vi "tm3samp_07b_dcimgrecorder_wVision.vi"() -> ()   [LabVIEW 2023]
panel:
  out "Frames Recorded":i32
  in  "Frames":i32=100
  in  "DCIMG Path":path
  out "Display":T1(plugin-control)
  out "DCAM Version":string
  out "Library Version":string
  out "Error Out":errorcluster {"code" format="%.0x"}
  # "This is an example of how to use the\nhard disk recorder functions to record\nimages to a DCIMG file, display images\nas you are recording,  and how to write\nmetadata to the file."
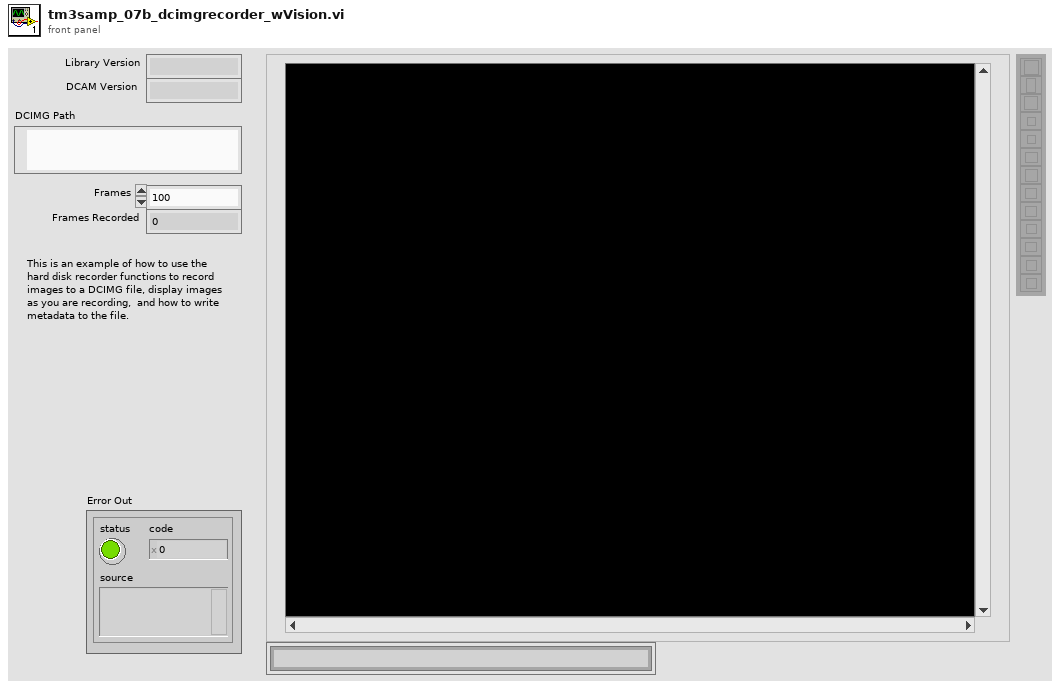
[diagram p1: front panel]
types:
  T1 = typedef "IMAQ Image.ctl" = refnum<image>
  T2 = cluster{"Capture Library":string, "DCAM-API":string}
  T3 = cluster{"Model":string, "Camera ID":string, "Firmware":string}
  T4 = cluster{"height":u32, "width":u32, "datatype":u32}
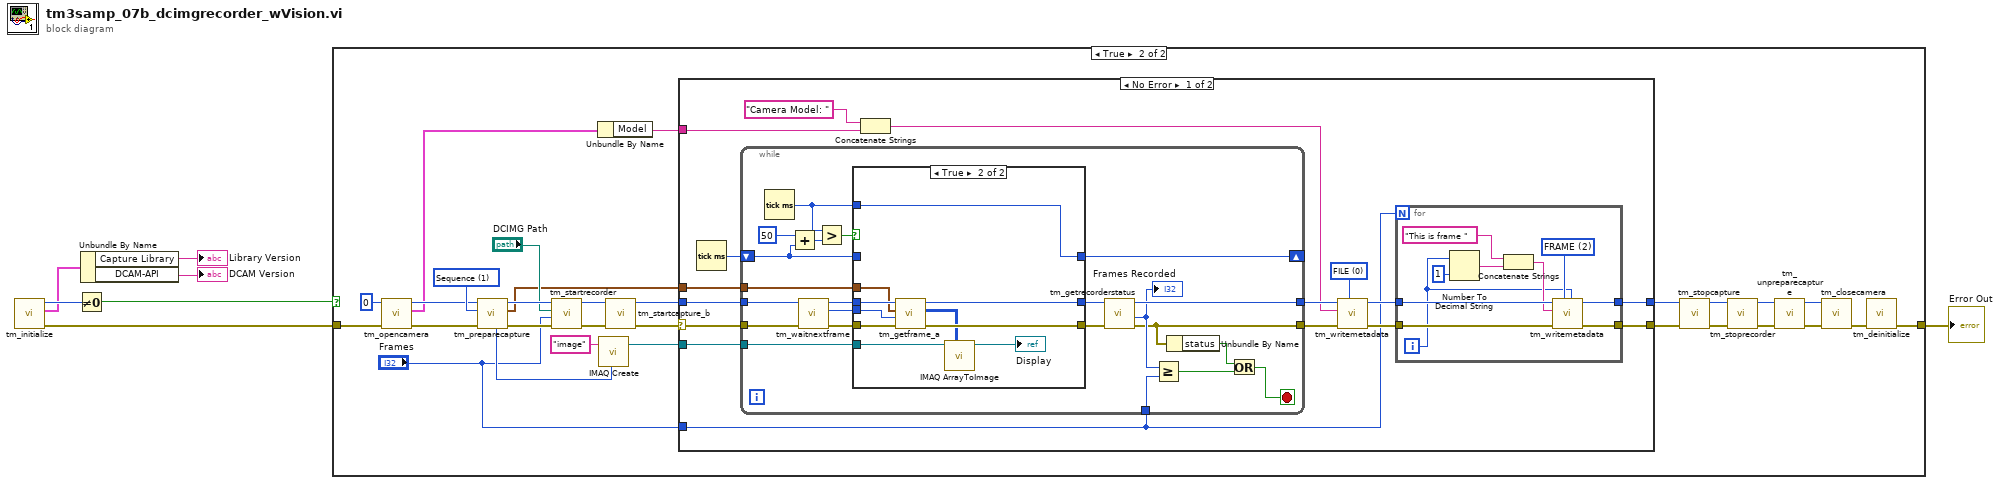
[diagram p0: block diagram]
diagram:
  n1 = call "tm_initialize.vi"() -> ("error out"=w4:errorcluster, "Version Info"=w3:T2, "Number Of Cameras"=w5:u32)  [unwired: 8 in, 1 out]
  n2 = Not Equal To 0?(x=w5) -> (x != 0?=w7:bool)
  n3 = Unbundle By Name(w3) -> ("Capture Library"=→"Library Version":string, "DCAM-API"=→"DCAM Version":string)
  n4 = case shown="True" w7 {
    tunnel: w4 -> [w8 w37]
    tunnel: [w8 w34] -> w6
    frame False {
    }
    frame True {
      w31 = 1 items=["Snap", "Sequence"] ("Capture mode")
      n5 = call "tm_opencamera.vi"("error in (no error)"=w37, "Camera Index"=u32 0) -> ("error out"=w29:errorcluster, "Camera Details"=w10:T3, "Handle out"=w30:u32)  [unwired: 7 in]
      n6 = call "tm_preparecapture.vi"("error in (no error)"=w29, "Capture mode"=w31, "Handle in"=w30) -> ("error out"=w26:errorcluster, "Buffer Info"=w16:T4, "Handle out"=w27:u32, "Image type"=w14:u32)  [unwired: 5 in]
      n7 = call "tm_startrecorder.vi"("error in (no error)"=w26, "frames"="Frames", "File"="DCIMG Path", "Handle in"=w27) -> ("error out"=w25:errorcluster, "Handle out"=w24:u32)  [unwired: 6 in]
      n8 = Unbundle By Name(w10) -> ("Model"=w9:string)
      n9 = call "IMAQ Create"("Image Name"="image", "Image Type"=w14) -> ("New Image"=w15:T1)  [unwired: 3 in, 1 out]
      n10 = call "tm_startcapture_b.vi"("error in (no error)"=w25, "Handle in"=w24) -> ("error out"=w18:errorcluster, "Handle out"=w17:u32)  [unwired: 8 in]
      n11 = case shown="No Error" w18 {
        selector: w18 -> [w52 w99]
        tunnel: w17 -> [w51 w100]
        tunnel: w16 -> [w50 _]
        tunnel: w15 -> [w49 _]
        tunnel: "Frames" -> [w38 _]
        tunnel: [w42 w100] -> w12
        tunnel: [w41 w99] -> w11
        tunnel: w9 -> [w40 _]
        frame No Error {
          w47 = 0 items=["FILE"=0, "FRAME"=2] ("Type")
          n12 = Tick Count (ms)() -> (millisecond timer value=w53:u32)
          n13 = while {
            tunnel: [w70] -> w43
            tunnel: [w67] -> w44
            tunnel: w50 -> [w74]
            tunnel: w51 -> [w84]
            tunnel: w52 -> [w85]
            shift-right: [w75] -> _
            shift-left: w53 -> [w76]
            tunnel: w49 -> [w73]
            tunnel: w38 -> [w68]
            stop <- w64 stop-if-true
            n14 = Tick Count (ms)() -> (millisecond timer value=w77:u32)
            n15 = Add(x=u32 50, y=w76) -> (x+y=w79:u32)
            n16 = call "tm_waitnextframe.vi"("error in (no error)"=w85, "Handle in"=w84) -> ("error out"=w82:errorcluster, "Frame Index"=w81:i32, "Handle out"=w83:u32)  [unwired: 6 in, 1 out]
            n17 = Greater?(x=w77, y=w79) -> (0:w78:bool)
            n18 = case shown="True" w78 {
              tunnel: w83 -> [w88 w98]
              tunnel: w82 -> [w87 w97]
              tunnel: w81 -> [_ w96]
              tunnel: w76 -> [w86 _]
              tunnel: w77 -> [_ w95]
              tunnel: [w88 w92] -> w72
              tunnel: [w87 w93] -> w71
              tunnel: [w86 w95] -> w75
              tunnel: w74 -> [_ w94]
              tunnel: w73 -> [_ w90]
              frame False {
              }
              frame True {
                n19 = call "tm_getframe_a.vi"("error in (no error)"=w97, "Frame Index"=w96, "Buffer Info"=w94, "Handle in"=w98) -> ("error out"=w93:errorcluster, "Data 16"=w91:u16[][], "Handle out"=w92:u32)  [unwired: 3 in, 2 out]
                n20 = call "IMAQ ArrayToImage"("Image Pixels (U16)"=w91, "Image"=w90) -> ("Image Out"=→"Display":T1)  [unwired: 8 in, 1 out]
              }
            }
            n21 = call "tm_getrecorderstatus.vi"("error in (no error)"=w71, "Handle"=w72) -> ("error out"=w67:errorcluster, "Count"=w69:i32, "Handle"=w70:u32)  [unwired: 6 in, 1 out]
            "Frames Recorded" <- w69
            n22 = Greater Or Equal?(x=w69, y=w68) -> (x >= y?=w65:bool)
            n23 = Unbundle By Name(w67) -> ("status"=w66:bool)
            n24 = Or(x=w66, y=w65) -> (x .or. y?=w64:bool)
          }
          n25 = Concatenate Strings("Camera Model: ", w40) -> (w39:string)
          n26 = call "tm_writemetadata.vi"("Type"=w47, "error in (no error)"=w44, "Metadata"=w39, "Handle"=w43) -> ("error out"=w46:errorcluster, "Handle"=w45:u32)  [unwired: 6 in]
          n27 = for {
            N: w38 -> [_]
            tunnel: w46 -> [w62]
            tunnel: w45 -> [w63]
            tunnel: [w55] -> w42
            tunnel: [w54] -> w41
            i -> [w56]
            w58 = 2 items=["FILE"=0, "FRAME"=2] ("Type")
            n28 = Number To Decimal String(number=w56, width (-)=i16 1) -> (decimal integer string=w60:string)
            n29 = Concatenate Strings("This is frame ", w60) -> (w59:string)
            n30 = call "tm_writemetadata.vi"("Index"=w56, "Type"=w58, "error in (no error)"=w62, "Metadata"=w59, "Handle"=w63) -> ("error out"=w54:errorcluster, "Handle"=w55:u32)  [unwired: 5 in]
          }
        }
        frame Error {
        }
      }
      n31 = call "tm_stopcapture.vi"("error in (no error)"=w11, "Handle in"=w12) -> ("error out"=w22:errorcluster, "Handle out"=w21:u32)  [unwired: 8 in]
      n32 = call "tm_stoprecorder.vi"("error in (no error)"=w22, "Handle in"=w21) -> ("error out"=w19:errorcluster, "Handle out"=w20:u32)  [unwired: 8 in]
      n33 = call "tm_unpreparecapture.vi"("error in (no error)"=w19, "Handle in"=w20) -> ("error out"=w33:errorcluster, "Handle out"=w32:u32)  [unwired: 8 in]
      n34 = call "tm_closecamera.vi"("error in (no error)"=w33, "Handle in"=w32) -> ("error out"=w35:errorcluster)  [unwired: 9 in]
      n35 = call "tm_deinitialize.vi"("error in (no error)"=w35) -> ("error out"=w34:errorcluster)  [unwired: 10 in]
    }
  }
  "Error Out" <- w6
